vi "ArrayTo1DI32.vi"(8 "ErrorIn(No Error)":errorcluster caption="entrée d'erreur (pas d'erreur)", 9 "Nombre":i32=-1, 10 "DelArrEnd":bool, 11 "tableau":i32[][](array[numeric])) -> (0 "sortie d'erreur":errorcluster, 2 "Size":i32, 3 "Array Out":i32[](array[numeric]))   [LabVIEW 2010]
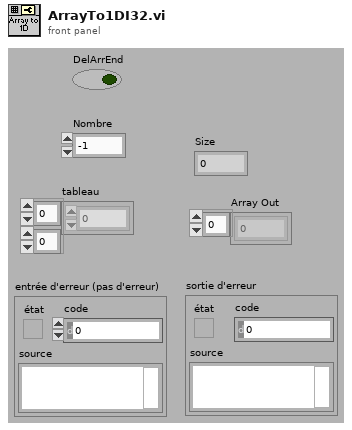
[diagram p1: front panel]
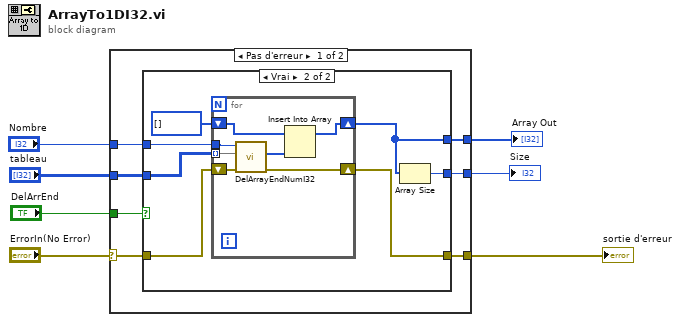
[diagram p0: block diagram]
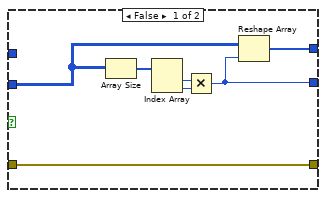
[diagram p2: hidden frame]
diagram:
  n1 = case shown="Pas d'erreur" "ErrorIn(No Error)" {
    selector: "ErrorIn(No Error)" -> [w10 w36]
    tunnel: [w9 w36] -> w6
    tunnel: "tableau" -> [w14 _]
    tunnel: [w13 _] -> w4
    tunnel: [w12 _] -> w3
    tunnel: "DelArrEnd" -> [w11 _]
    tunnel: "Nombre" -> [w8 _]
    frame No Error {
      n2 = case shown="Vrai" w11 {
        tunnel: w14 -> [w21 w28]
        tunnel: [w20 w23] -> w13
        tunnel: [w19 w22] -> w12
        tunnel: w10 -> [w15 w27]
        tunnel: [w15 w26] -> w9
        tunnel: w8 -> [_ w25]
        frame False {
          n3 = Array Size(array=w21) -> (size(s)=w18:i32[])
          n4 = Index Array(array=w18) -> (element #1=w16:i32, element #2=w17:i32)  [unwired: 2 in]
          n5 = Multiply(x=w16, y=w17) -> (x*y=w20:i32)
          n6 = Reshape Array(w21, w20) -> (w19:i32[])
        }
        frame True {
          n7 = for {
            tunnel: w28 -> [w35] mode=indexing
            shift-right: [w33] -> w26
            shift-left: w27 -> [w34]
            tunnel: w25 -> [w32]
            shift-right: [w29] -> w22
            shift-left: i32[] [] ("tableau") -> [w30]
            n8 = call <userlib>:"DelArrayEndNumI32.vi"("ErrorIn(No Error)"=w34, "Array In"=w35, "Nombre"=w32) -> ("sortie d'erreur"=w33:errorcluster, "Array Out"=w31:i32[])  [unwired: 7 in]
            n9 = Insert Into Array(array=w30, new element=w31) -> (w29:i32[])  [unwired: 1 in]
          }
          n10 = Array Size(array=w22) -> (size(s)=w23:i32)
        }
      }
    }
    frame Error {
    }
  }
  "sortie d'erreur" <- w6
  "Size" <- w4
  "Array Out" <- w3
